vi "borrar_bloqueo.vi"   [LabVIEW 2009]
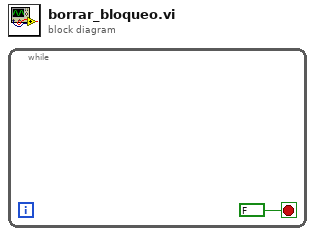
[diagram p0: block diagram]
diagram:
  n1 = while {
    stop <- FALSE stop-if-true
  }
